vi "Set Oval Diameter.vi"(9 "ROI Diameter":i32, 11 "Oval Points in":i32[](array[numeric])) -> (3 "Circle Points out":i32[](array[numeric]))   [LabVIEW 2021, in "Image.lvlib"]
uses:
  Image.lvlib
  Math/Math.lvlib
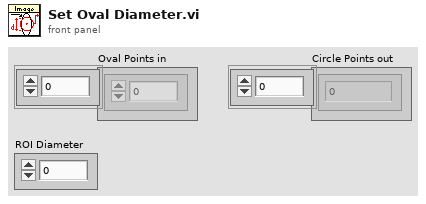
[diagram p1: front panel]
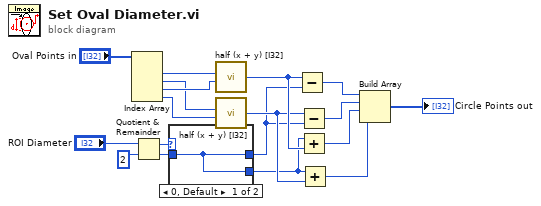
[diagram p0: block diagram]
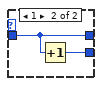
[diagram p2: hidden frame]
diagram:
  n1 = Index Array(array="Oval Points in") -> (element #1=w11:i32, element #2=w8:i32, element #3=w10:i32, element #4=w7:i32)  [unwired: 4 in]
  n2 = Quotient & Remainder(x="ROI Diameter", y=2) -> (x-y*floor(x/y)=w4:i32, floor(x/y)=w3:i32)
  n3 = case shown="0, Default" w4 {
    tunnel: w3 -> [w19 w21]
    tunnel: [w19 w21] -> w2
    tunnel: [w19 w20] -> w1
    frame 0, Default {
    }
    frame 1 {
      n4 = Increment(x=w21) -> (x+1=w20:i32)
    }
  }
  n5 = call "half (x + y) [I32].vi"("y"=w10, "x"=w11) -> ("(x+y)/2"=w9:i32)  [unwired: 4 in]
  n6 = call "half (x + y) [I32].vi"("y"=w7, "x"=w8) -> ("(x+y)/2"=w6:i32)  [unwired: 4 in]
  n7 = Subtract(x=w9, y=w2) -> (x-y=w13:i32)
  n8 = Subtract(x=w6, y=w2) -> (x-y=w14:i32)
  n9 = Add(x=w1, y=w9) -> (x+y=w15:i32)
  n10 = Add(x=w1, y=w6) -> (x+y=w16:i32)
  n11 = Build Array(w13, w14, w15, w16) -> (→"Circle Points out":i32[])
